vi "Build VIPB.vi"(6 "Buildlog":path, 7 "Build number":u32, 8 "error in":errorcluster, 10 "args":string[](array[string]), 11 "VIP Path":path) -> (0 "error out":errorcluster)   [LabVIEW 2010]
uses:
  <vilib>/JKI/VIPM API/VIPM API_vipm_api.lvlib
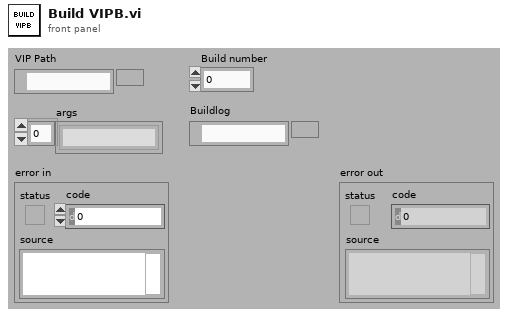
[diagram p1: front panel]
types:
  T1 = typedef "VIPM API_vipm_api.lvlib/VI Package Build Spec Data Cluster_vipm_api.ctl" = cluster{"Package Version":T2, "Product Name":string, "Company Name":string, "Author Name (Person or Company)":string, "Product Homepage (URL)":string, "Legal Copyright":string, "License Agreement Name":string, "Product Description Summary":string, "Product Description":string, "Release Notes - Change Log":string}
  T2 = typedef "VIPM API_vipm_api.lvlib/Version Info Cluster_vipm_api.ctl" = cluster{"major":u32, "minor":u32, "patch":u32, "build":u32}
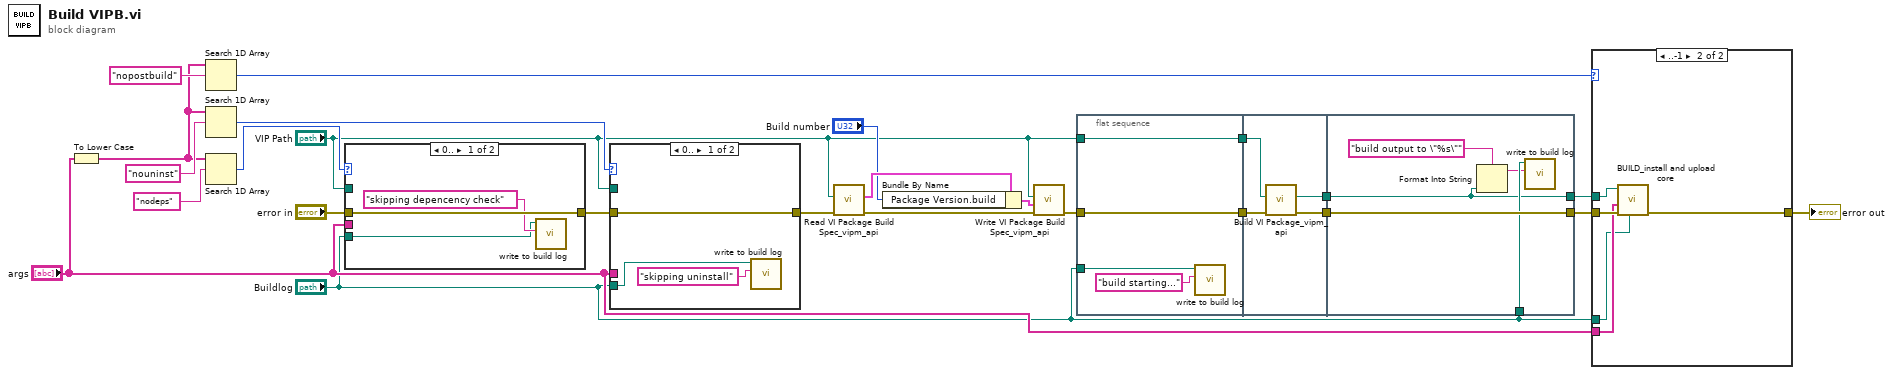
[diagram p0: block diagram]
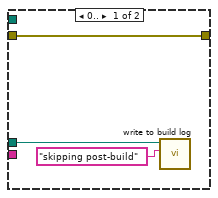
[diagram p2: hidden frame]
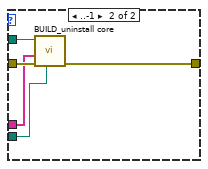
[diagram p3: hidden frame]
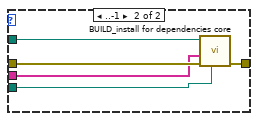
[diagram p4: hidden frame]
diagram:
  n1 = To Lower Case(string="args") -> (all lower case string=w8:string[])
  n2 = Search 1D Array(1D array=w8, element="nopostbuild") -> (index of element=w7:i32)  [unwired: 1 in]
  n3 = Search 1D Array(1D array=w8, element="nouninst") -> (index of element=w16:i32)  [unwired: 1 in]
  n4 = Search 1D Array(1D array=w8, element="nodeps") -> (index of element=w19:i32)  [unwired: 1 in]
  n5 = case shown="0.." w19 {
    tunnel: [w28 w32] -> w17
    tunnel: "error in" -> [w28 w33]
    tunnel: "VIP Path" -> [_ w31]
    tunnel: "Buildlog" -> [w26 w30]
    tunnel: "args" -> [_ w29]
    frame 0.. {
      n6 = call "write to build log.vi"("text"="skipping depencency check", "log"=w26) -> ()  [unwired: 10 in]
    }
    frame ..-1 {
      n7 = call "BUILD_install for dependencies core.vi"("buildlog"=w30, "error in"=w33, "args"=w29, "vipb path"=w31) -> ("error out"=w32:errorcluster)  [unwired: 7 in]
    }
  }
  n8 = case shown="0.." w16 {
    tunnel: [w36 w39] -> w15
    tunnel: w17 -> [w36 w41]
    tunnel: "VIP Path" -> [_ w40]
    tunnel: "Buildlog" -> [w34 w38]
    tunnel: "args" -> [_ w37]
    frame 0.. {
      n9 = call "write to build log.vi"("text"="skipping uninstall", "log"=w34) -> ()  [unwired: 10 in]
    }
    frame ..-1 {
      n10 = call "BUILD_uninstall core.vi"("Buildlog"=w38, "error in"=w41, "args"=w37, "appended path"=w40) -> ("error out"=w39:errorcluster)  [unwired: 7 in]
    }
  }
  n11 = call <vilib>:"Read VI Package Build Spec_vipm_api.vi"("error in (no error)"=w15, "Path to VIPB File"="VIP Path") -> ("error out"=w22:errorcluster, "VI Package Build Spec Data"=w25:T1)  [unwired: 8 in]
  n12 = Bundle By Name(cluster=w25, "Package Version.build"="Build number") -> (w23:T1)
  n13 = call <vilib>:"Write VI Package Build Spec_vipm_api.vi"("error in (no error)"=w22, "VI Package Build Spec Data"=w23, "Path to VIPB File"="VIP Path") -> ("error out"=w21:errorcluster)  [unwired: 8 in]
  n14 = flat-sequence {
    tunnel: "VIP Path" -> [w44]
    tunnel: w21 -> [w45]
    tunnel: [w45] -> w6
    tunnel: [w44] -> w5
    tunnel: "Buildlog" -> [w42]
    tunnel: w6 -> [w49]
    tunnel: w5 -> [w47]
    tunnel: [w48] -> w4
    tunnel: [w46] -> w1
    tunnel: [w54] -> w13
    tunnel: w4 -> [w54]
    tunnel: "Buildlog" -> [w53]
    tunnel: [w51] -> w2
    tunnel: w1 -> [w51]
    frame #0 {
      n15 = call "write to build log.vi"("text"="build starting...", "log"=w42) -> ()  [unwired: 10 in]
    }
    frame #1 {
      n16 = call <vilib>:"Build VI Package_vipm_api.vi"("error in (no error)"=w49, "Path to VIPB File"=w47) -> ("error out"=w48:errorcluster, "Build Output"=w46:path)  [unwired: 8 in]
    }
    frame #2 {
      n17 = Format Into String(format string="build output to \"%s\"", w51) -> (resulting string=w52:string)  [unwired: 2 in, 1 out]
      n18 = call "write to build log.vi"("text"=w52, "log"=w53) -> ()  [unwired: 10 in]
    }
  }
  n19 = case shown="..-1" w7 {
    tunnel: w13 -> [w57 w62]
    tunnel: [w57 w61] -> w12
    tunnel: "args" -> [_ w60]
    tunnel: "Buildlog" -> [w55 w59]
    tunnel: w2 -> [_ w58]
    frame 0.. {
      n20 = call "write to build log.vi"("text"="skipping post-build", "log"=w55) -> ()  [unwired: 10 in]
    }
    frame ..-1 {
      n21 = call "BUILD_install and upload core.vi"("Buildlog"=w59, "error in"=w62, "args"=w60, "vip built path"=w58) -> ("error out"=w61:errorcluster)  [unwired: 7 in]
    }
  }
  "error out" <- w12
